vi "Write NewCommand.vi"(8 "error in (no error)":errorcluster, 10 "Command.lvclass":refnum<class "Command.lvclass">, 11 "System in":refnum<class "System.lvclass">) -> (0 "error out":errorcluster, 3 "System out":refnum<class "System.lvclass">)   [LabVIEW 2013, in "System.lvclass"]
uses:
  System.lvclass
  Commands/Command/Command.lvclass
  System.lvclass/System.ctl
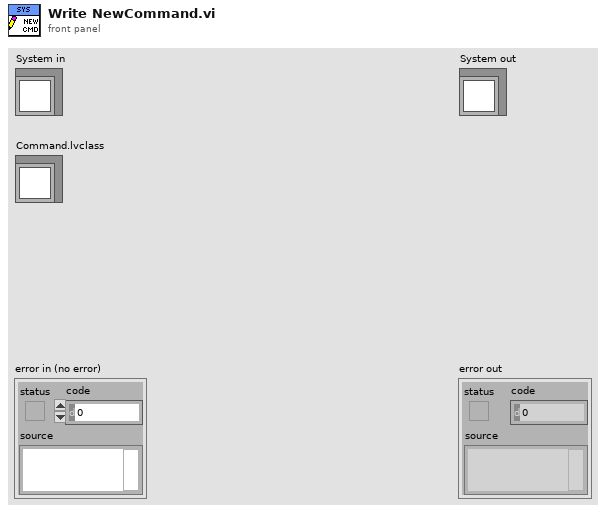
[diagram p1: front panel]
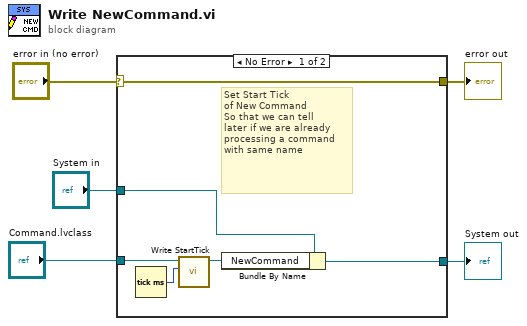
[diagram p0: block diagram]
diagram:
  n1 = case shown="No Error" "error in (no error)" {
    selector: "error in (no error)" -> [w11 w12]
    tunnel: [w11 w12] -> w4
    tunnel: [w9 w13] -> w2
    tunnel: "System in" -> [w10 w13]
    tunnel: "Command.lvclass" -> [w8 _]
    frame No Error {
      # "Set Start Tick\nof New Command\nSo that we can tell \nlater if we are already \nprocessing a command \nwith same name"
      n2 = Tick Count (ms)() -> (millisecond timer value=w6:u32)
      n3 = call-dynamic "Write StartTick.vi"("StartTick"=w6, "Command in"=w8) -> ("Command out"=w7:refnum<class "Command.lvclass">)  [unwired: 8 in, 1 out]
      n4 = Bundle By Name(cluster=w10, "NewCommand"=w7) -> (w9:refnum<class "System.lvclass">)
    }
    frame Error {
    }
  }
  "error out" <- w4
  "System out" <- w2
